vi "testFlattenPressureToXML.vi"() -> ()   [LabVIEW 2012, in "UnitsAndXML.lvlib"]
uses:
  <userlib>/Common/UnitsAndXML/UnitsAndXML.lvlib
  <userlib>/Common/UnitsAndXML/FlattenItemWithUnitToXML/FlattenPressureToXML/PressureUnit.ctl
  <userlib>/Common/UnitsAndXML/FlattenItemWithUnitToXML/FlattenPressureToXML/typeMethods/flattenPressureToXML_Array.vi
  <userlib>/Common/UnitsAndXML/FlattenItemWithUnitToXML/FlattenPressureToXML/typeMethods/flattenPressureToXML_Scalar.vi
panel:
  out "error out":errorcluster
  in  "pressureUnitInXML":T1
  out "xmlStringArray":string
  out "xmlStringScalar":string
  in  "pressure":dbl[unit][](array[numeric])=[1519874.9999999998, 3039749.9999999995, 4559625.0, 6079499.999999999]
  in  "pressure":dbl[unit]=1519874.9999999998
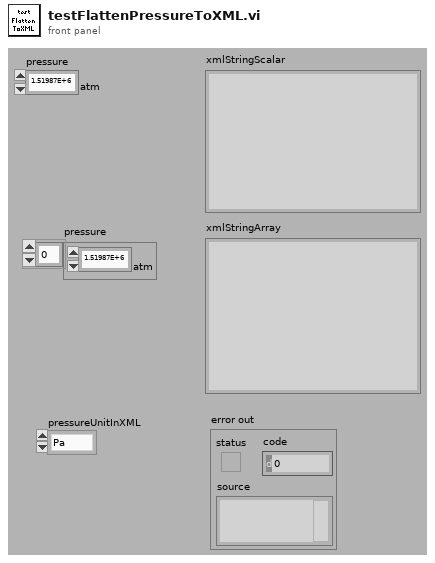
[diagram p1: front panel]
types:
  T1 = typedef "UnitsAndXML.lvlib/PressureUnit.ctl" = enum16{"Pa", "atm", "bar", "mbar", "m.Hg", "psi", "torr"}
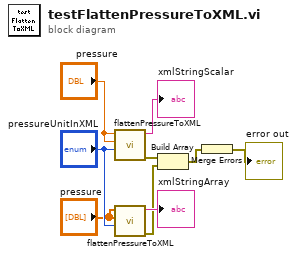
[diagram p0: block diagram]
diagram:
  n1 = call-poly <userlib>:"flattenPressureToXML.vi"("pressureUnitInXML"="pressureUnitInXML", "pressureAgain"="pressure", "pressure"="pressure") -> ("error out"=w6:errorcluster, "xmlString"=→"xmlStringScalar":string)  [unwired: 7 in]
  n2 = call-poly <userlib>:"flattenPressureToXML.vi"("pressureUnitInXML"="pressureUnitInXML", "pressureAgain"="pressure", "pressure"="pressure") -> ("error out"=w1:errorcluster, "xmlString"=→"xmlStringArray":string)  [unwired: 7 in]
  n3 = Build Array(w6, w1) -> (w7:errorcluster[])
  n4 = Merge Errors(w7) -> (→"error out":errorcluster)
